vi "process-booleans_sysID.vi"(10 "boolean indicators 2":T1) -> (0 "scaning finished":bool, 2 "boolean indicators":T1)   [LabVIEW 2017]
uses:
  controls/boolean_info.ctl
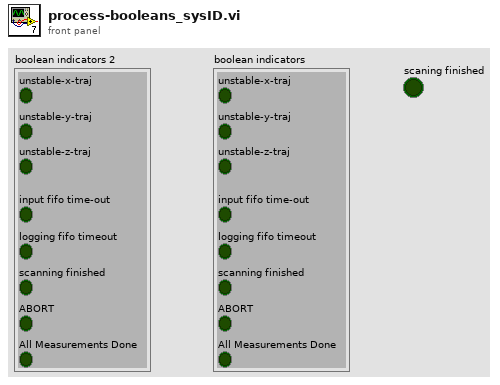
[diagram p1: front panel]
types:
  T1 = typedef "boolean_info.ctl" = cluster{"unstable-z-traj":bool, "input fifo time-out":bool, "logging fifo timeout":bool, "scanning finished":bool, "unstable-x-traj":bool, "unstable-y-traj":bool, "ABORT":bool, "All Measurements Done":bool}
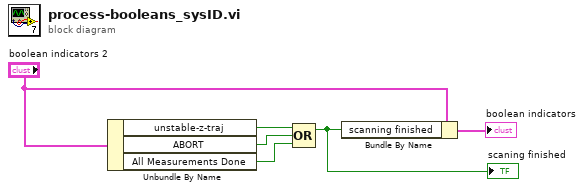
[diagram p0: block diagram]
diagram:
  n1 = Unbundle By Name("boolean indicators 2") -> ("unstable-z-traj"=w6:bool, "ABORT"=w2:bool, "All Measurements Done"=w1:bool)
  n2 = Compound Arithmetic op=OR(w6, w2, w1) -> (w5:bool)
  "scaning finished" <- w5
  n3 = Bundle By Name(cluster="boolean indicators 2", "scanning finished"=w5) -> (→"boolean indicators":T1)
